vi "Down Reset.vi"() -> ()   [LabVIEW 2019]
uses:
  Implementation/Arm Operations.ctl
  Implementation/Arm Setpoints.ctl
  <vilib>/Rock Robotics/WPI/Framework/Completion Status.ctl
  <vilib>/Rock Robotics/WPI/Framework/Completion Notifier.ctl
  <vilib>/Rock Robotics/WPI/Framework/Command Status Info.ctl
panel:
  in  "Description":string
  out "Command Info Out":T1
  in  "Command Info In":T1
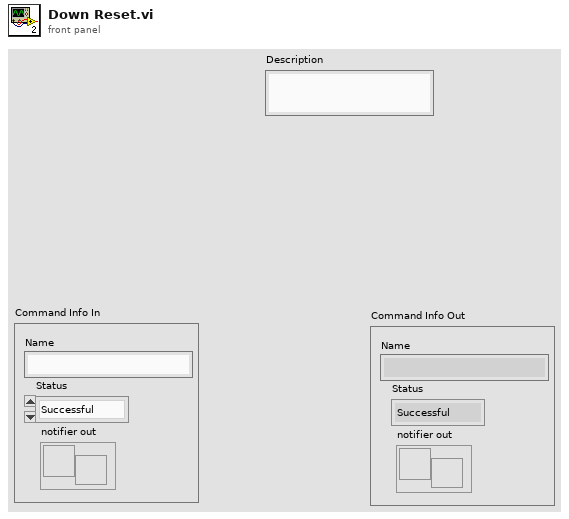
[diagram p1: front panel]
types:
  T1 = typedef "Command Status Info.ctl" = cluster{"Name":string, "Status":T2, "notifier out":T3}
  T2 = typedef "Completion Status.ctl" = enum16{"Successful", "Aborted", "Incomplete"}
  T3 = typedef "Completion Notifier.ctl" = refnum<notifier>
  T4 = typedef "Arm Setpoints.ctl" = cluster{"Operation":T5, "Degrees":dbl}
  T5 = typedef "Arm Operations.ctl" = enum16{"Reserve", "Read Current", "bore_test", "Up", "Down", "Up Reset", "Down Reset", "Immediate", ""}
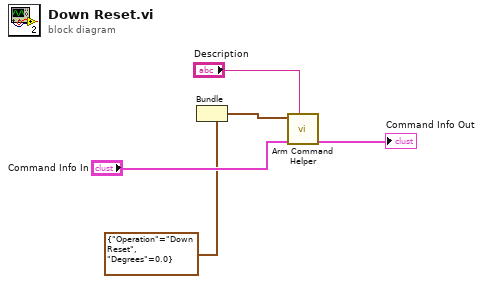
[diagram p0: block diagram]
diagram:
  n1 = Bundle(cluster=T4 {"Operation"=enum."Down Reset", "Degrees"=0.0} ("SubSystem Data")) -> (w1:T4)  [unwired: 2 in]
  n2 = call "Arm Command Helper.vi"("Description"="Description", "Command Info In"="Command Info In", "SubSystem Data"=w1) -> ("Command Info Out"=→"Command Info Out":T1)  [unwired: 6 in, 2 out]
